vi "PutCluster.vi"(8 "error in (no error)":errorcluster, 10 "Cluster":variant, 11 "MsgPackSerializer in":refnum<class "MsgPackSerializer.lvclass">) -> (0 "error out":errorcluster, 3 "MsgPackSerializer out":refnum<class "MsgPackSerializer.lvclass">)   [LabVIEW 2015, in "MsgPackSerializer.lvclass"]
uses:
  MsgPackSerializer.lvclass
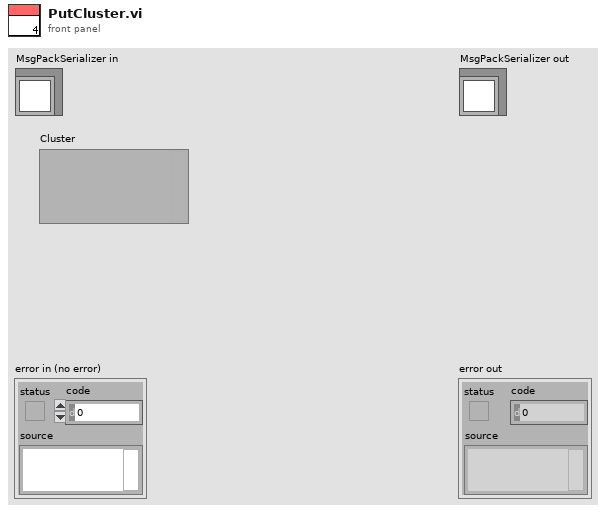
[diagram p1: front panel]
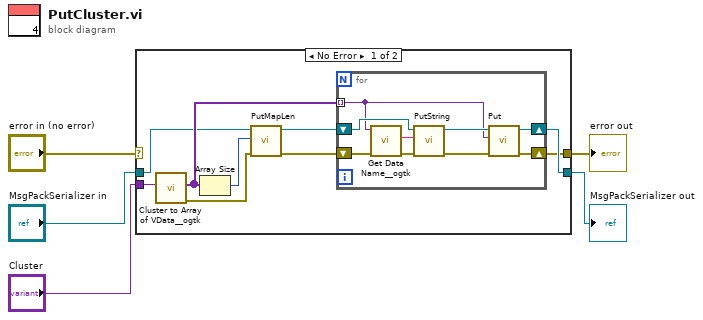
[diagram p0: block diagram]
diagram:
  n1 = case shown="No Error" "error in (no error)" {
    selector: "error in (no error)" -> [_ w25]
    tunnel: [w7 w25] -> w4
    tunnel: [w8 w24] -> w2
    tunnel: "MsgPackSerializer in" -> [w12 w24]
    tunnel: "Cluster" -> [w13 _]
    frame No Error {
      n2 = call <userlib>:"Cluster to Array of VData__ogtk.vi"("Cluster"=w13) -> ("error out"=w11:errorcluster, "Array of VData"=w14:variant[])  [unwired: 9 in]
      n3 = Array Size(array=w14) -> (size(s)=w6:i32)
      n4 = call "PutMapLen.vi"("error in (no error)"=w11, "len"=w6, "MsgPackSerializer in"=w12) -> ("error out"=w9:errorcluster, "MsgPackSerializer out"=w10:refnum<class "MsgPackSerializer.lvclass">)  [unwired: 7 in]
      n5 = for {
        shift-right: [w15] -> w7
        shift-left: w9 -> [w23]
        tunnel: w14 -> [w18] mode=indexing
        shift-right: [w17] -> w8
        shift-left: w10 -> [w21]
        n6 = call <userlib>:"Get Data Name__ogtk.vi"("error in (no error)"=w23, "Data"=w18) -> ("error out"=w19:errorcluster, "Data Name"=w22:string)  [unwired: 7 in, 1 out]
        n7 = call "PutString.vi"("error in (no error)"=w19, "string"=w22, "MsgPackSerializer in"=w21) -> ("error out"=w16:errorcluster, "MsgPackSerializer out"=w20:refnum<class "MsgPackSerializer.lvclass">)  [unwired: 7 in]
        n8 = call "Put.vi"("error in (no error)"=w16, "Data"=w18, "MsgPackSerializer in"=w20) -> ("error out"=w15:errorcluster, "MsgPackSerializer out"=w17:refnum<class "MsgPackSerializer.lvclass">)  [unwired: 7 in]
      }
    }
    frame Error {
    }
  }
  "error out" <- w4
  "MsgPackSerializer out" <- w2
